vi "Write output range.vi"(8 "error in (no error)":errorcluster, 10 "output range":cluster{"output high":dbl, "output low":dbl}={"output high"=100.0, "output low"=-100.0} {"output low" format="%.2f"; "output high" format="%.2f"}, 11 "PID in":refnum<class "PID.lvclass">) -> (0 "error out":errorcluster, 3 "PID out":refnum<class "PID.lvclass">)   [LabVIEW 2024, in "PID.lvlib" / "PID.lvclass"]
uses:
  PID.lvclass
  PID.lvclass/PID.ctl
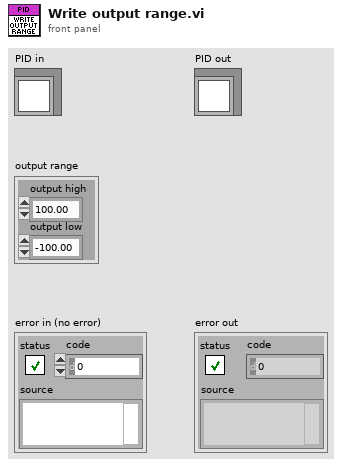
[diagram p1: front panel]
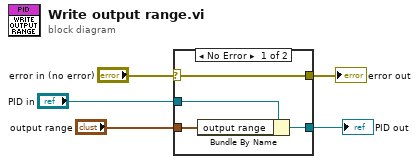
[diagram p0: block diagram]
diagram:
  n1 = case shown="No Error" "error in (no error)" {
    selector: "error in (no error)" -> [w9 w10]
    tunnel: [w9 w10] -> w4
    tunnel: [w7 w11] -> w2
    tunnel: "PID in" -> [w8 w11]
    tunnel: "output range" -> [w6 _]
    frame No Error {
      n2 = Bundle By Name(cluster=w8, "output range"=w6) -> (w7:refnum<class "PID.lvclass">)
    }
    frame Error {
    }
  }
  "error out" <- w4
  "PID out" <- w2
